vi "Find XML Descriptor.vi"(8 "error in":errorcluster, 11 "Project Path":path) -> (0 "error out":errorcluster, 2 "Found ?":bool, 3 "XML Path":path, 5 "Custom Device Name":string, 7 "Common Doc Dir":string)   [LabVIEW 2019, in "LVLIBP CD XML Updater.lvlib" / "Project XML Editor.lvclass"]
uses:
  Project XML Editor.lvclass
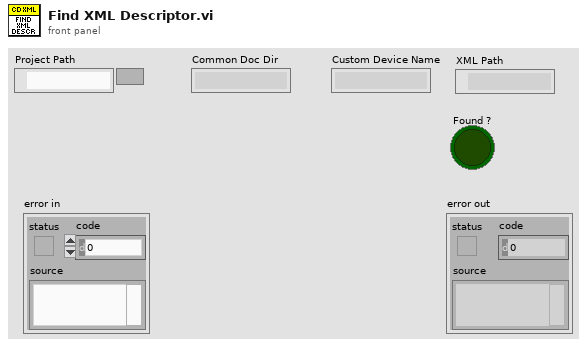
[diagram p1: front panel]
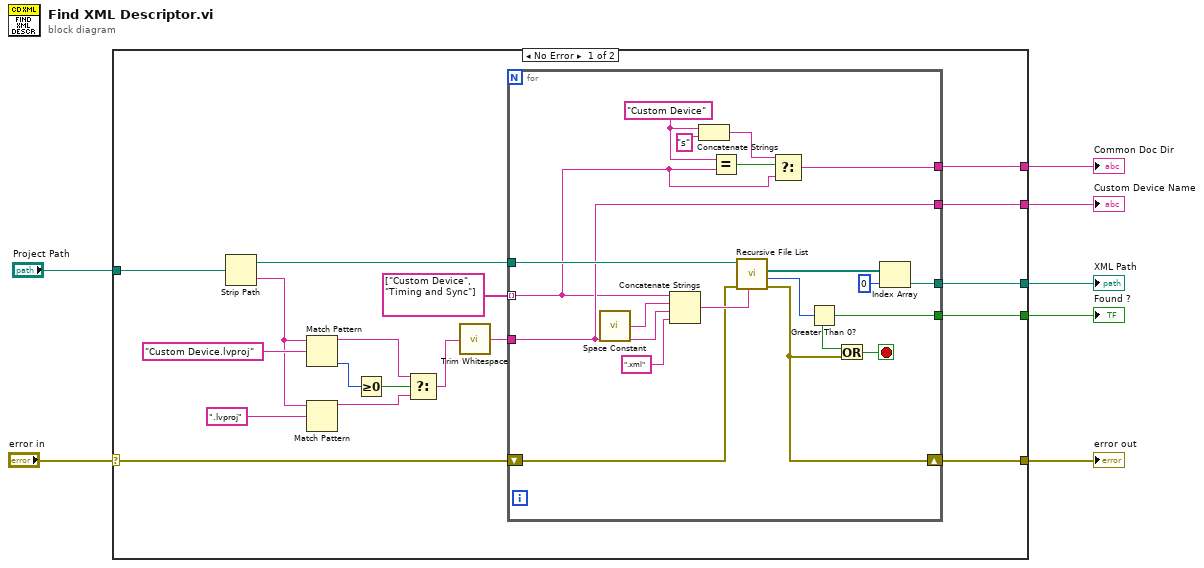
[diagram p0: block diagram]
diagram:
  n1 = case shown="No Error" "error in" {
    selector: "error in" -> [w19 w45]
    tunnel: "Project Path" -> [w21 _]
    tunnel: [w20 _] -> w6
    tunnel: [w18 w45] -> w4
    tunnel: [w17 _] -> w3
    tunnel: [w16 _] -> w2
    tunnel: [w15 _] -> w1
    frame No Error {
      n2 = Strip Path(path=w21) -> (stripped path=w23:path, name=w13:string)
      n3 = Match Pattern(string=w13, regular expression="Custom Device.lvproj") -> (before substring=w10:string, offset past match=w12:i32)  [unwired: 1 in, 2 out]
      n4 = Match Pattern(string=w13, regular expression=".lvproj") -> (before substring=w8:string)  [unwired: 1 in, 3 out]
      n5 = Greater Or Equal To 0?(x=w12) -> (x >= 0?=w11:bool)
      n6 = Select(t=w10, s=w11, f=w8) -> (s? t:f=w9:string)
      n7 = call <vilib>:"Trim Whitespace.vi"("string"=w9) -> ("trimmed string"=w25:string)  [unwired: 1 in]
      n8 = for {
        tunnel: w23 -> [w42]
        tunnel: string[] ["Custom Device", "Timing and Sync"] -> [w27] mode=indexing
        tunnel: w25 -> [w32]
        tunnel: [w36] -> w20
        tunnel: [w35] -> w17
        shift-right: [w33] -> w18
        shift-left: w19 -> [w34]
        tunnel: [w32] -> w16
        tunnel: [w26] -> w15
        stop <- w39 stop-if-true
        w30 = "Custom Device" ("y")
        n9 = call <vilib>:"Space Constant.vi"() -> ("String"=w43:string)
        n10 = Concatenate Strings(w27, w43, w32, ".xml" ("string")) -> (w41:string)
        n11 = Concatenate Strings(w30, "s" ("string")) -> (w28:string)
        n12 = Equal?(x=w30, y=w27) -> (x = y?=w31:bool)
        n13 = call <vilib>:"Recursive File List.vi"("pattern"=w41, "error in (no error)"=w34, "Folder Path"=w42) -> ("error out"=w33:errorcluster, "Number of Files"=w40:i32, "All Files in Dir"=w38:path[])  [unwired: 4 in, 2 out]
        n14 = Select(t=w28, s=w31, f=w27) -> (s? t:f=w26:string)
        n15 = Greater Than 0?(x=w40) -> (x > 0?=w35:bool)
        n16 = Or(x=w35, y=w33) -> (x .or. y?=w39:bool)
        n17 = Index Array(array=w38, index=0) -> (element=w36:path)
      }
    }
    frame Error {
    }
  }
  "XML Path" <- w6
  "error out" <- w4
  "Found ?" <- w3
  "Custom Device Name" <- w2
  "Common Doc Dir" <- w1
